vi "Get Song Progress Info.vi"(8 "error in (no error)":errorcluster, 11 "Song in":refnum<class "Song.lvclass">) -> (0 "error out":errorcluster, 1 "Percent Complete":dbl, 2 "Time Remaining (s)":T1 format="%<%M:%S>T", 3 "Song out":refnum<class "Song.lvclass">, 4 "Complete?":bool, 5 "Time Complete (s)":dbl)   [LabVIEW 2015, in "Song.lvclass"]
uses:
  Song.lvclass
  Song Duration.ctl
  Song.lvclass/Song.ctl
  Read Duration (s).vi
  Read Play Index (s).vi
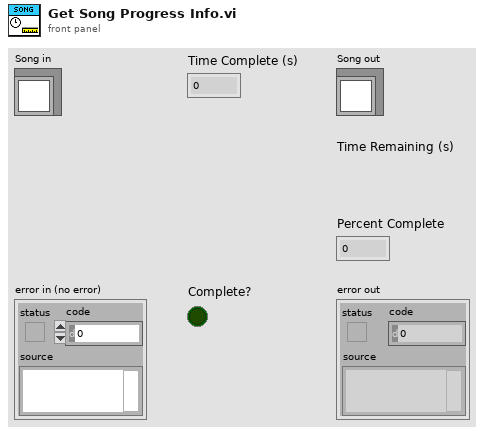
[diagram p1: front panel]
types:
  T1 = typedef "Song.lvclass/Song Duration.ctl" = timestamp
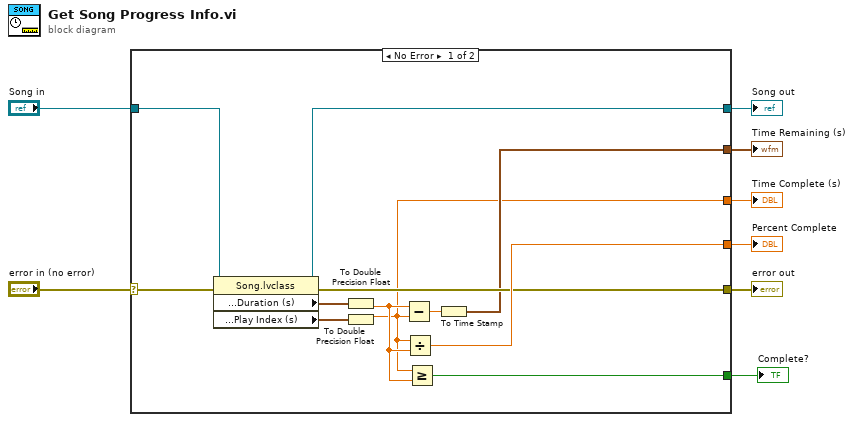
[diagram p0: block diagram]
diagram:
  n1 = case shown="No Error" "error in (no error)" {
    selector: "error in (no error)" -> [w20 w22]
    tunnel: [w14 w22] -> w7
    tunnel: [w18 w21] -> w5
    tunnel: "Song in" -> [w19 w21]
    tunnel: [w15 _] -> w4
    tunnel: [w12 _] -> w3
    tunnel: [w10 _] -> w2
    tunnel: [w9 _] -> w1
    frame No Error {
      n2 = property class="Song.lvclass"(reference=w19, error in=w20) -> (reference out=w18:refnum<class "Song.lvclass">, error out=w14:errorcluster, "API:Data Member Accessors:Duration (s)"=w17:T1, "API:Data Member Accessors:Play Index (s)"=w16:T1)
      n3 = To Double Precision Float(number=w17) -> (double precision float=w11:dbl)
      n4 = To Double Precision Float(number=w16) -> (double precision float=w10:dbl)
      n5 = Subtract(x=w11, y=w10) -> (x-y=w13:dbl)
      n6 = Divide(x=w10, y=w11) -> (x/y=w15:dbl)
      n7 = Greater Or Equal?(x=w10, y=w11) -> (x >= y?=w9:bool)
      n8 = To Time Stamp(1:w13) -> (0:w12:timestamp)
    }
    frame Error {
    }
  }
  "error out" <- w7
  "Song out" <- w5
  "Percent Complete" <- w4
  "Time Remaining (s)" <- w3
  "Time Complete (s)" <- w2
  "Complete?" <- w1
